vi "Do.vi"(8 "error in (no error)":errorcluster, 10 "Actor in":refnum<class "Actor.lvclass">, 11 "Update Monitored Datum Msg":refnum<class "Update Monitored Datum Msg.lvclass">) -> (0 "error out":errorcluster, 2 "Actor out":refnum<class "Actor.lvclass">)   [LabVIEW 2017, in "Update Monitored Datum Msg.lvclass"]
doc: "(<B>Filename</B>: Actor Framework.lvlib:Message.lvclass:Do.vi)\n\nDefines what a message does when it is received by an actor. Generally, a message instructs an actor to invoke one of its methods. By default, this method does nothing. A child class must override it to define behavior. Create a child class by using the Actor Framework Message Maker dialog box."
uses:
  Update Monitored Datum Msg.lvclass
  C:/Git/mva-framework/gpm_packages/@cs/transport/Source/Concrete/ActorMessageTransport/Notification Msg/Notification Msg.lvclass
  <vilib>/ActorFramework/Actor/Actor.lvclass
  ListboxBusMonitorPanel/ListboxBusMonitorPanel.lvclass
  C:/Program Files (x86)/National Instruments/LabVIEW 2017/vi.lib/ActorFramework/Actor/Actor.lvclass
  gpm_packages/@cs/transport/Source/Concrete/ActorMessageTransport/Notification Msg/Notification Msg.lvclass/Notification Msg.ctl
  gpm_packages/@cs/transport/Source/Concrete/ActorMessageTransport/Notification Msg/Notification Msg.lvclass
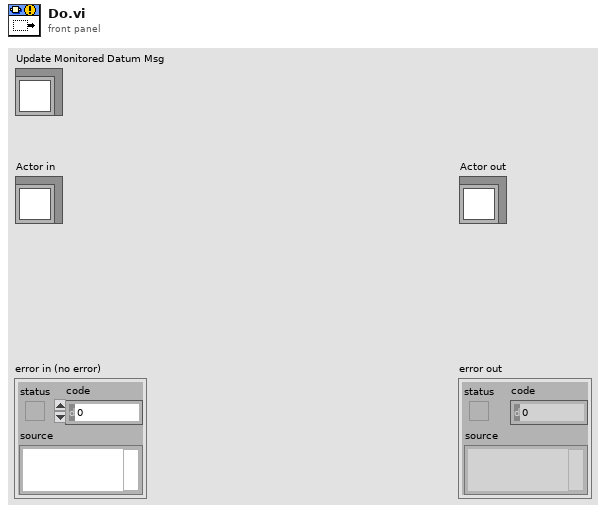
[diagram p1: front panel]
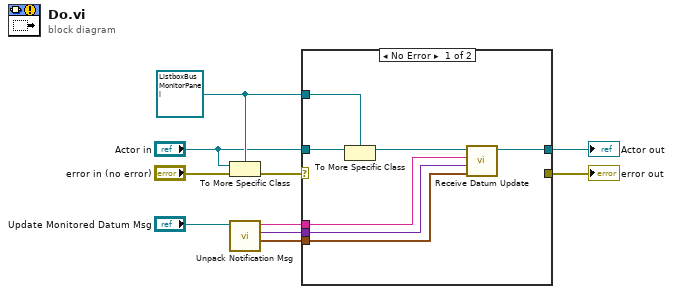
[diagram p0: block diagram]
diagram:
  w9 = refnum<class "ListboxBusMonitorPanel.lvclass"> refnum ("Actor in")
  n1 = To More Specific Class(target class=w9, reference="Actor in", error in="error in (no error)") -> (error out=w10:errorcluster)  [unwired: 1 out]
  n2 = call "Unpack Notification Msg.vi"("Notification Msg"="Update Monitored Datum Msg") -> ("Publication Time"=w1:timestamp, "Value"=w2:variant, "Datum Name"=w3:string)  [unwired: 8 in]
  n3 = case shown="No Error" w10 {
    selector: w10 -> [_ w19]
    tunnel: [_ w19] -> w5
    tunnel: [w17 w18] -> w6
    tunnel: "Actor in" -> [w16 w18]
    tunnel: w9 -> [w15 _]
    tunnel: w3 -> [w13 _]
    tunnel: w2 -> [w12 _]
    tunnel: w1 -> [w11 _]
    frame No Error {
      n4 = To More Specific Class(target class=w15, reference=w16) -> (specific class reference=w14:refnum<class "ListboxBusMonitorPanel.lvclass">)  [unwired: 1 in, 1 out]
      n5 = call "Receive Datum Update.vi"("Publication Time"=w11, "Value"=w12, "Datum Name"=w13, "ListboxBusMonitorPanel in"=w14) -> ("ListboxBusMonitorPanel out"=w17:refnum<class "ListboxBusMonitorPanel.lvclass">)  [unwired: 7 in]
    }
    frame Error {
      # "If type check fails, pass the\noriginal object out again."
    }
  }
  "error out" <- w5
  "Actor out" <- w6
